vi "Subset Status.vi"(8 "error in (no error)":errorcluster, 9 "count (1)":u64=1, 10 "group index":u64, 11 "Transfer Group Status in":refnum<class "Transfer Group Status.lvclass">) -> (0 "error out":errorcluster, 1 "index + count":u64, 2 "subset Transfer Group Status":refnum<class "Transfer Group Status.lvclass">, 3 "Transfer Group Status out":refnum<class "Transfer Group Status.lvclass">)   [LabVIEW 2017, in "DSF Core.lvlib" / "Transfer Group Status.lvclass"]
uses:
  Transfer Group Status.lvclass
  C:/Program Files (x86)/National Instruments/LabVIEW 2017/vi.lib/NI/Memory Manager/Classes/Pointer/Pointer.lvclass
  DSF Configuration API/Public/Controls/DSF Transfer Group Status.ctl
  <vilib>/NI/Memory Manager/Classes/Pointer/Pointer.lvclass/Pointer.ctl
  29846c0c-ce60-4e1a-a9dd-72c3b6361b89.vi
  <vilib>/NI/Memory Manager/Classes/Pointer/Get Address.vi
  <vilib>/NI/Memory Manager/Classes/Pointer/Encapsulate.vi
  <vilib>/NI/Memory Manager/Classes/Pointer/Check Null Pointer.vi
  <vilib>/NI/Memory Manager/Classes/Pointer/Check Length.vi
  <vilib>/NI/Memory Manager/Classes/Pointer/Set Size.vi
  <vilib>/NI/Memory Manager/Classes/Pointer/Set Address.vi
  <vilib>/NI/Memory Manager/Classes/Pointer/Set Internal.vi
  <vilib>/NI/Memory Manager/Classes/Pointer/Errors.vi
  <vilib>/NI/Memory Manager/Classes/Pointer/Null Pointer.vi
  <vilib>/NI/Memory Manager/Classes/Pointer/Is Null.vi
  <vilib>/NI/Memory Manager/Classes/Pointer/Get Size.vi
  <vilib>/NI/Memory Manager/Classes/Pointer/Check Pointer Bounds.vi
  <vilib>/NI/Memory Manager/Classes/Pointer/Create Error.vi
  <vilib>/NI/Memory Manager/Classes/Pointer/Out of Bounds.vi
  <vilib>/NI/Memory Manager/VIs/New Error Cluster Constant.vi
  <vilib>/NI/Memory Manager/VIs/New Error Cluster Constant (512B).vi
  <vilib>/NI/Memory Manager/VIs/Error Cluster.Set Status.vi
  <vilib>/NI/Memory Manager/VIs/Error Cluster.Set Code.vi
  <vilib>/NI/Memory Manager/VIs/Error Cluster.Set VI Source.vi
  <vilib>/NI/Memory Manager/Constants/Constants.vi
  <vilib>/NI/Memory Manager/Constants/Library Name.vi
  <vilib>/NI/Memory Manager/Classes/Pointer/Pointer Error Info.vi
  <vilib>/NI/Memory Manager/VIs/Source.Write.String.vi
  <vilib>/NI/Memory Manager/Constants/Pointer Class Name.vi
  <vilib>/NI/Memory Manager/Classes/Pointer/Write Pointer Size.vi
  <vilib>/NI/Memory Manager/VIs/Source.Write.Scalar.Base10.vi
  <vilib>/NI/Memory Manager/VIs/Source.Write.Scalar.Base10 (U64).vi
  <vilib>/NI/Memory Manager/Classes/Pointer/Pointer.lvclass
  DSF Core.lvlib
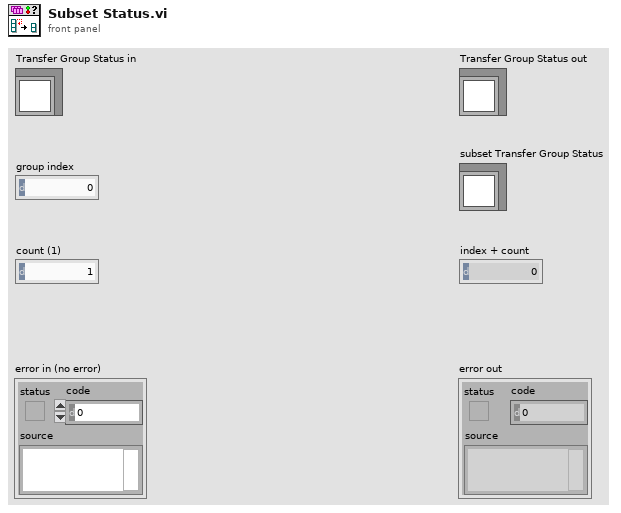
[diagram p1: front panel]
types:
  T1 = typedef "DSF Core.lvlib/DSF Transfer Group Status.ctl" = cluster{"late count":u64, "iteration":u64}
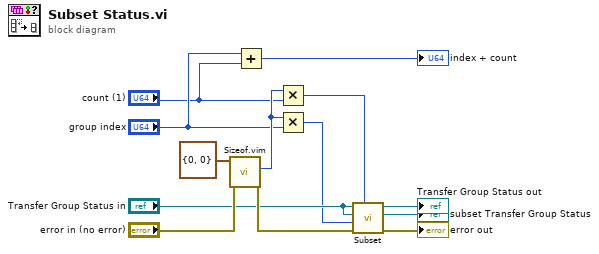
[diagram p0: block diagram]
diagram:
  n1 = call "Sizeof.vim"("error in (no error)"="error in (no error)", "anything"=T1 {"late count"=0, "iteration"=0} ("Transfer Group status")) -> ("error out"=w13:errorcluster, "size"=w5:u64)  [unwired: 8 in]
  n2 = Add(x="group index", y="count (1)") -> (x+y=→"index + count":u64)
  n3 = Multiply(x=w5, y="count (1)") -> (x*y=w6:u64)
  n4 = Multiply(x=w5, y="group index") -> (x*y=w4:u64)
  n5 = call <vilib>:"Subset.vi"("length (-1: rest)"=w6, "error in (no error)"=w13, "offset (0)"=w4, "subset Pointer type"="Transfer Group Status in", "base Pointer in"="Transfer Group Status in") -> ("error out"=→"error out":errorcluster, "subset Pointer"=→"subset Transfer Group Status":refnum<class "Transfer Group Status.lvclass">, "base Pointer out"=→"Transfer Group Status out":refnum<class "Transfer Group Status.lvclass">)  [unwired: 3 in, 1 out]
